vi "LogScaleImage.vi"(2 "A/D bits":u16, 3 "input array":dbl[][](array[numeric])) -> (1 "log scale image":dbl[][](array[numeric]))   [LabVIEW 2022 SP3]
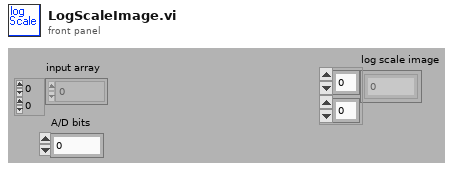
[diagram p1: front panel]
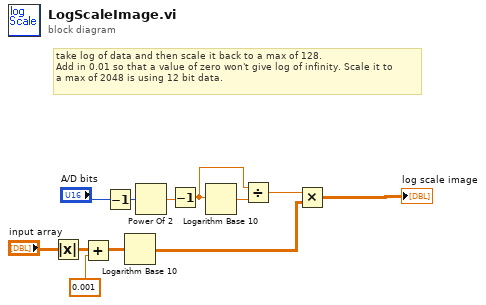
[diagram p0: block diagram]
diagram:
  # "take log of data and then scale it back to a max of 128.\nAdd in 0.01 so that a value of zero won't give log of infinity. Scale it to\na max of 2048 is using 12 bit data."
  n1 = Absolute Value(x="input array") -> (abs(x)=w2:dbl[][])
  n2 = Add(x=w2, y=0.001) -> (x+y=w12:dbl[][])
  n3 = Decrement(x="A/D bits") -> (x-1=w8:u16)
  n4 = Logarithm Base 10(1:w12) -> (0:w9:dbl[][])
  n5 = Power Of 2(x=w8) -> (2^x=w7:dbl)
  n6 = Decrement(x=w7) -> (x-1=w5:dbl)
  n7 = Logarithm Base 10(1:w5) -> (0:w6:dbl)
  n8 = Divide(x=w5, y=w6) -> (x/y=w4:dbl)
  n9 = Multiply(x=w4, y=w9) -> (x*y=→"log scale image":dbl[][])
